vi "Thingworx_ParseBrackets.vi"(1 "body":string) -> (0 "In Brackets":string[](array[string]))   [LabVIEW 2019]
panel:
  out "start":i32[](array[numeric])
  out "Numeric":i32
  out "end":i32[](array[numeric])
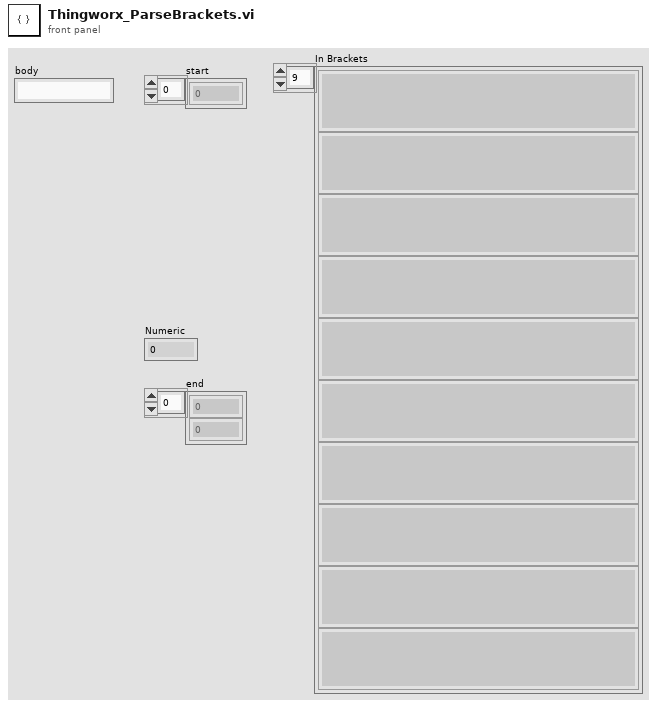
[diagram p1: front panel]
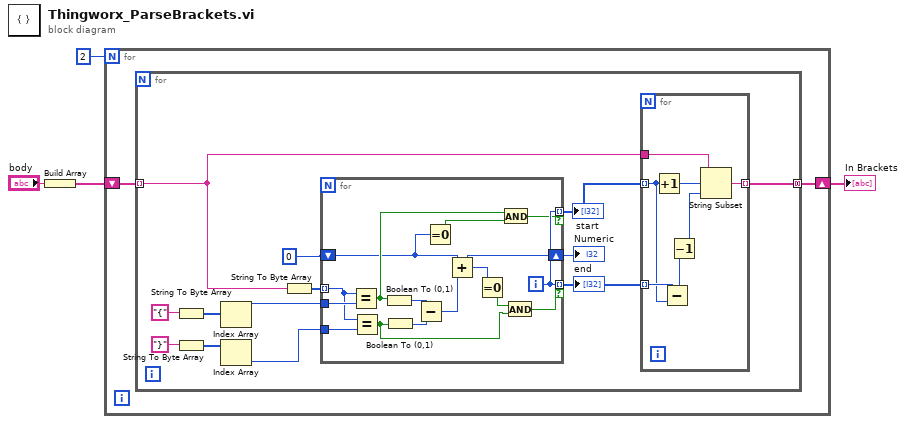
[diagram p0: block diagram]
diagram:
  n1 = Build Array("body") -> (w2:string[])
  n2 = for {
    N: 2 -> [_]
    shift-right: [w5] -> w4
    shift-left: w2 -> [w6]
    n3 = for {
      tunnel: w6 -> [w10] mode=indexing
      tunnel: [w7] -> w5 mode=concatenating
      n4 = String To Byte Array(string="{" ("regular expression")) -> (unsigned byte array=w17:u8[])
      n5 = String To Byte Array(string="}" ("regular expression")) -> (unsigned byte array=w16:u8[])
      n6 = Index Array(array=w17) -> (element=w13:u8)  [unwired: 1 in]
      n7 = Index Array(array=w16) -> (element=w12:u8)  [unwired: 1 in]
      n8 = String To Byte Array(string=w10) -> (unsigned byte array=w19:u8[])
      n9 = for {
        tunnel: w19 -> [w40] mode=indexing
        shift-right: [w35] -> w11
        shift-left: 0 -> [w28]
        tunnel: w13 -> [w41]
        tunnel: w12 -> [w39]
        tunnel: [w30] -> w8 mode=indexing if=w33
        tunnel: [w30] -> w9 mode=indexing if=w29
        i -> [w30]
        n10 = Equal?(x=w40, y=w41) -> (x = y?=w32:bool)
        n11 = Equal?(x=w40, y=w39) -> (x = y?=w34:bool)
        n12 = Boolean To (0,1)(Boolean=w32) -> (0, 1=w37:i16)
        n13 = Boolean To (0,1)(Boolean=w34) -> (0, 1=w38:i16)
        n14 = Subtract(x=w37, y=w38) -> (x-y=w36:i16)
        n15 = Equal To 0?(x=w28) -> (x = 0?=w27:bool)
        n16 = Add(x=w28, y=w36) -> (x+y=w35:i32)
        n17 = Equal To 0?(x=w35) -> (x = 0?=w31:bool)
        n18 = And(x=w32, y=w27) -> (x .and. y?=w29:bool)
        n19 = And(x=w31, y=w34) -> (x .and. y?=w33:bool)
      }
      "end" <- w8
      "Numeric" <- w11
      "start" <- w9
      n20 = for {
        tunnel: w10 -> [w26]
        tunnel: w9 -> [w24] mode=indexing
        tunnel: w8 -> [w25] mode=indexing
        tunnel: [w22] -> w7 mode=indexing
        n21 = Increment(x=w24) -> (x+1=w21:i32)
        n22 = Subtract(x=w25, y=w24) -> (x-y=w23:i32)
        n23 = Decrement(x=w23) -> (x-1=w20:i32)
        n24 = String Subset(string=w26, offset (0)=w21, length (rest)=w20) -> (substring=w22:string)
      }
    }
  }
  "In Brackets" <- w4
